vi "ImageInitStage.vi"(0 "Image in":refnum<class "Image.lvclass">, 7 "data queue":refnum<queue>, 9 "Stage Data queue":refnum<queue>, 12 "error in (no error)":errorcluster) -> (4 "Image out":refnum<class "Image.lvclass">, 15 "error out":errorcluster)   [LabVIEW 2012, in "Image.lvclass"]
uses:
  classes/Image.lvclass
  classes/Image.lvclass/Image.ctl
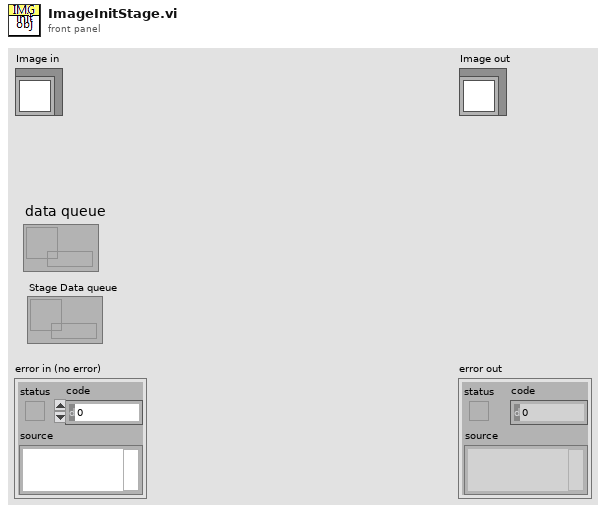
[diagram p1: front panel]
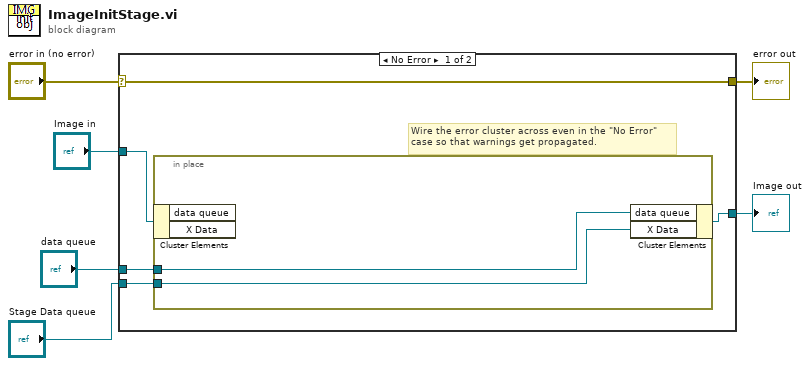
[diagram p0: block diagram]
diagram:
  n1 = case shown="No Error" "error in (no error)" {
    selector: "error in (no error)" -> [w11 w15]
    tunnel: [w11 w15] -> w5
    tunnel: [w9 w14] -> w3
    tunnel: "Image in" -> [w10 w14]
    tunnel: "data queue" -> [w8 _]
    tunnel: "Stage Data queue" -> [w7 _]
    frame No Error {
      # "Wire the error cluster across even in the \"No Error\"\ncase so that warnings get propagated."
      n2 = in-place {
        in-place-border: w8 -> [w13]
        in-place-border: w7 -> [w12]
        n3 = in-place-cluster #1(w10) -> ()  [unwired: 2 out]
        n4 = in-place-cluster #1("data queue"=w13, "X Data"=w12) -> (w9:refnum<class "Image.lvclass">)
      }
    }
    frame Error {
    }
  }
  "error out" <- w5
  "Image out" <- w3
